vi "Load or Create Group.vi"(8 "error in (no error)":errorcluster, 10 "Write Pref":refnum<user-event>, 11 "Group Name":string) -> (0 "error out":errorcluster, 3 "Pref Group":refnum<class "Pref Group.lvclass">, 5 "Config Manager":refnum<class "Config Manager.lvclass">)   [LabVIEW 2023, in "User Prefs.lvlib" / "PrefsDB.lvclass"]
uses:
  PrefsDB.lvclass
  Pref Group/Pref Group.lvclass
  lv-cdm/CDM-Config/Config Manager/Config Manager.lvclass
  Write Pref Data.ctl
  lv-promises/Promises/Promise/Promise.lvclass
  lv-cdm/CDM-Config/Config-JSON/Config-JSON.lvclass
  PrefsDB.lvclass/PrefsDB.ctl
  lv-cdm/CDM-Config/Config Storage/Config Storage.lvclass
  User Prefs.lvlib
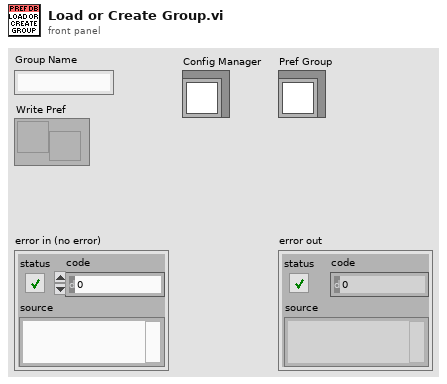
[diagram p1: front panel]
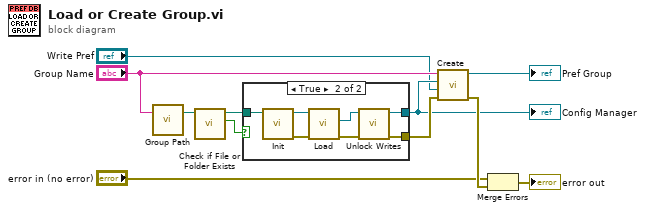
[diagram p0: block diagram]
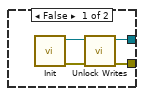
[diagram p2: hidden frame]
diagram:
  n1 = call "Group Path.vi"("Group Name"="Group Name") -> ("Group Path"=w9:path)  [unwired: 6 in]
  n2 = call <vilib>:"Check if File or Folder Exists.vi"("path"=w9) -> ("file or folder exists?"=w8:bool, "dup path"=w7:path)  [unwired: 8 in, 1 out]
  n3 = case shown="True" w8 {
    tunnel: w7 -> [_ w22]
    tunnel: [w12 w16] -> w5
    tunnel: [w14 w17] -> w10
    frame False {
      n4 = call "Init.vi"() -> ("error out"=w15:errorcluster, "Config Manager out"=w13:refnum<class "Config Manager.lvclass">)  [unwired: 10 in]
      n5 = call "Unlock Writes.vi"("error in (no error)"=w15, "Config Manager in"=w13) -> ("error out"=w14:errorcluster, "Config Manager out"=w12:refnum<class "Config Manager.lvclass">)  [unwired: 8 in]
    }
    frame True {
      n6 = call "Init.vi"("Path"=w22) -> ("error out"=w20:errorcluster, "Config-JSON out"=w21:refnum<class "Config-JSON.lvclass">)  [unwired: 9 in]
      n7 = call "Load.vi"("error in (no error)"=w20, "Config Storage in"=w21) -> ("error out"=w18:errorcluster, "Config"=w19:refnum<class "Config Manager.lvclass">)  [unwired: 7 in, 1 out]
      n8 = call "Unlock Writes.vi"("error in (no error)"=w18, "Config Manager in"=w19) -> ("error out"=w17:errorcluster, "Config Manager out"=w16:refnum<class "Config Manager.lvclass">)  [unwired: 8 in]
    }
  }
  "Config Manager" <- w5
  n9 = call "Create.vi"("error in (no error)"=w10, "Write Pref"="Write Pref", "Config Manager"=w5, "Group"="Group Name") -> ("error out"=w11:errorcluster, "Pref Group out"=→"Pref Group":refnum<class "Pref Group.lvclass">)  [unwired: 6 in]
  n10 = Merge Errors("error in (no error)", w11) -> (→"error out":errorcluster)
